vi "Main Global.vi"() -> ()   [LabVIEW 2017]
panel:
  out "New Calcs Done":bool
  out "Subtraction Result":dbl
  out "Multiplication Result":dbl
  out "Division Result":dbl
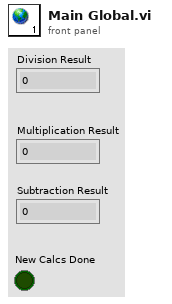
[diagram p1: front panel]
diagram:
